vi "Main.vi"() -> ()   [LabVIEW 2019]
uses:
  Typedefs/#enum_State.ctl
  <vilib>/sound2/lvsound2.llb/Sound Data Format.ctl
  <vilib>/sound2/lvsound2.llb/Sampling Mode.ctl
  Typedefs/#cluster_ApplicationData.ctl
  <vilib>/sound2/lvsound2.llb/Sound File Refnum.ctl
  <vilib>/sound2/lvsound2.llb/Sound Input Task ID.ctl
  <vilib>/Utility/sysdir.llb/System Directory Type.ctl
  <vilib>/sound2/lvsound2.llb/Sound Input Read (DBL).vi
panel:
  out "Raw Data":waveform(dbl)[](graph)
  out "Spectrum Data":cluster{"f0":dbl, "df":dbl, "magnitude":dbl[]}[](graph)
  out "Threshold Exceeded?":bool
  in  "Threshold, dB":dbl=-100.0 format="%#_13g"
  in  "Upper Fc":dbl=3500.0 format="%#_13g"
  in  "Lower Fc":dbl=300.0 format="%#_13g"
  in  "Order":i32=6
  in  "Type":T1(ring)
  in  "Stop":bool
  # "FILTER SETTINGS"
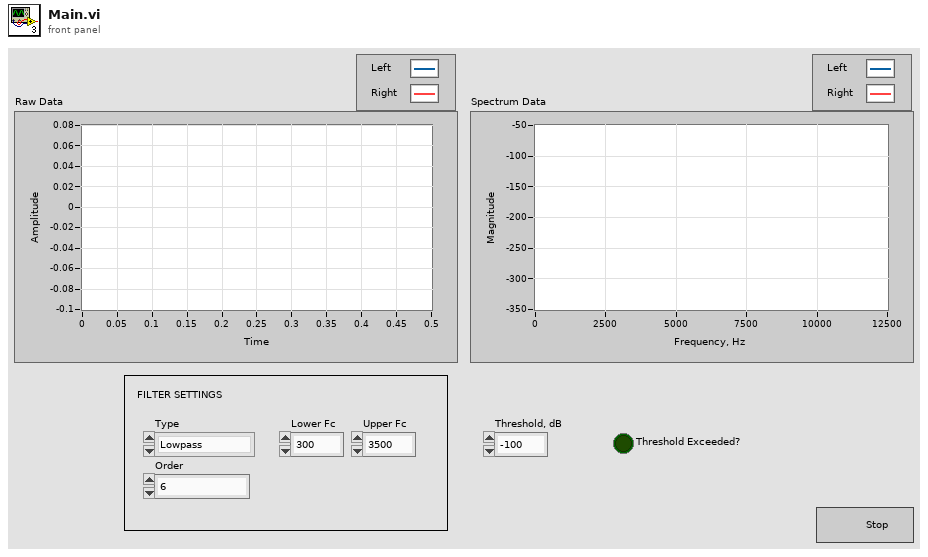
[diagram p1: front panel]
types:
  T1 = enum16{"Lowpass", "Highpass", "Bandpass", "Bandstop"}
  T2 = typedef "#enum_State.ctl" = enum16{"Init", "Acquisition", "Error Handler", "Exit"}
  T3 = enum16{"open", "replace", "create", "open or create", "replace or create", "replace or create with confirmation"}
  T4 = typedef "Sound Data Format.ctl" = cluster{"sample rate (S/s)":dbl, "number of channels":i32, "bits per sample":i32}
  T5 = typedef "#cluster_ApplicationData.ctl" = cluster{"Sound file refnum":T6, "Acquisition task ID":T7, "Sound format":T4, "Number of samples/channel":i32, "Logging file refnum":refnum<file>}
  T6 = typedef "Sound File Refnum.ctl" = refnum<file>
  T7 = typedef "Sound Input Task ID.ctl" = u32
  T8 = typedef "System Directory Type.ctl" = i32
  T9 = typedef "Sampling Mode.ctl" = i32
  T10 = cluster{"Topology":enum16{"Off", "Butterworth", "Chebyshev", "Inverse Chebyshev", "Elliptic", "Bessel"}, "Type":enum16{"Lowpass", "Highpass", "Bandpass", "Bandstop"}, "Order":i32, "Lower Fc":dbl, "Upper Fc":dbl, "PB Ripple":dbl, "SB Attenuation":dbl}
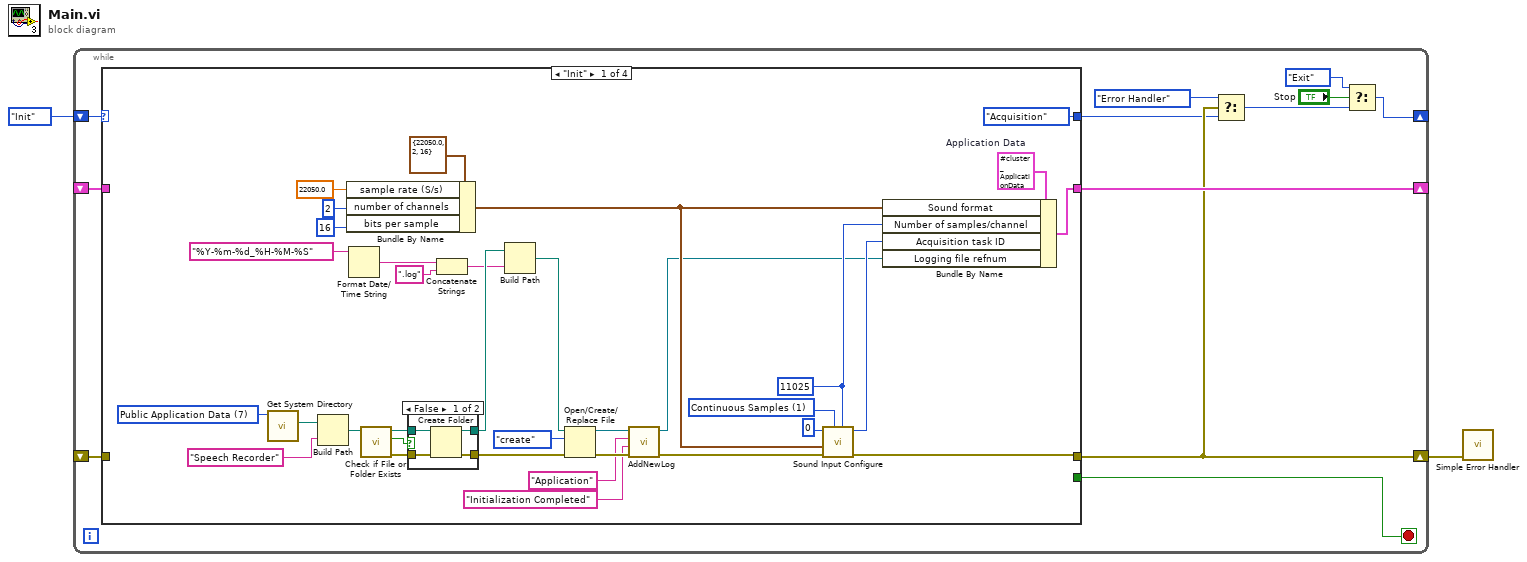
[diagram p0: block diagram]
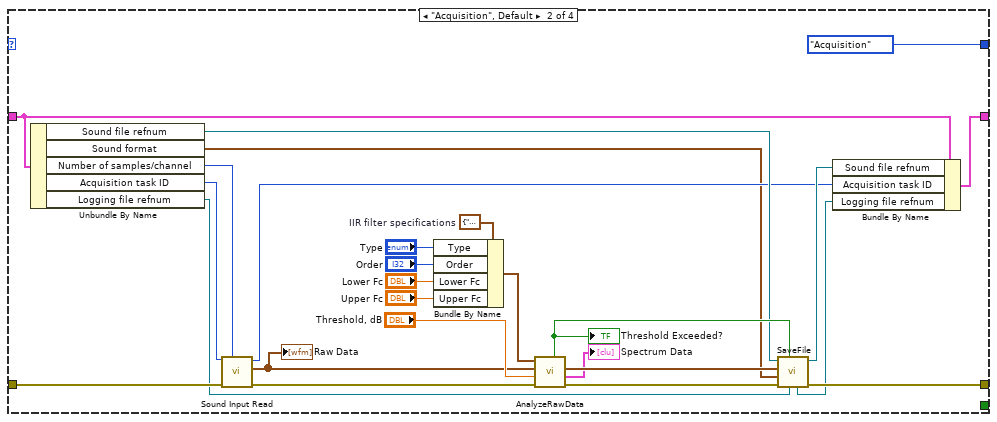
[diagram p3: hidden frame]
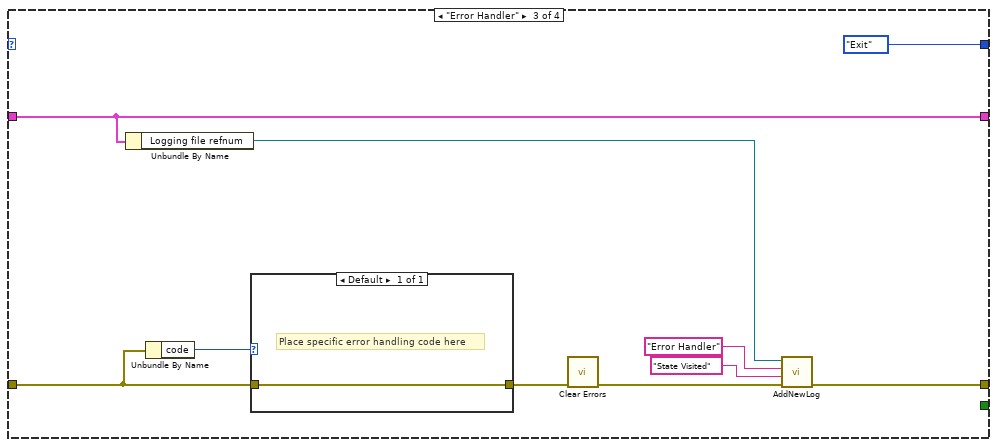
[diagram p4: hidden frame]
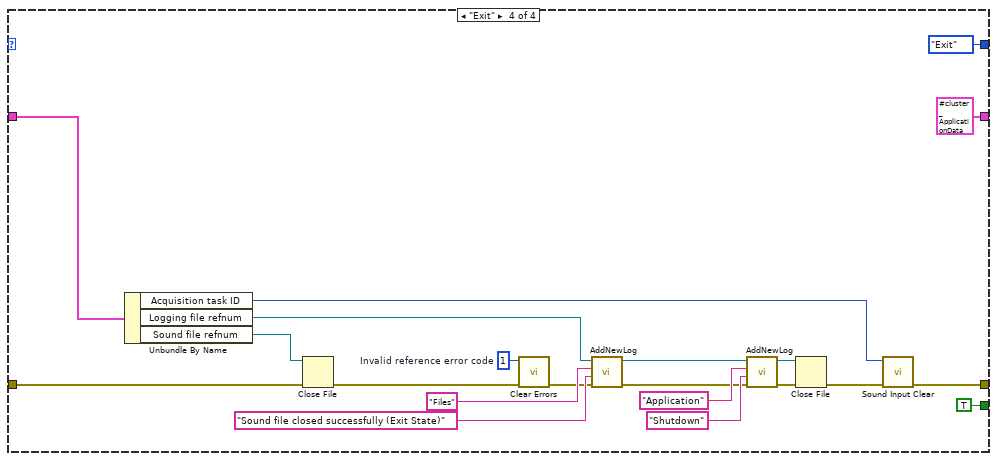
[diagram p5: hidden frame]
diagram:
  n1 = while {
    shift-right: [w5] -> _
    shift-left: #enum_State."Init" ("State") -> [w14]
    shift-right: [w12] -> _
    shift-left: _ -> [w13]
    shift-right: [w9] -> w2
    shift-left: _ -> [w11]
    stop <- w10 stop-if-true
    n2 = case shown="\"Init\"" w14 {
      tunnel: w11 -> [_ w80 w81 w112]
      tunnel: [w40 w67 w88 w95] -> w9
      tunnel: w13 -> [_ w64 w85 w109]
      tunnel: [w41 w63 w85 T5 {"Sound file refnum"=refnum, "Acquisition task ID"=0, "Sound format"={"sample rate (S/s)"=22050.0, "number of channels"=2, "bits per sample"=16}, "Number of samples/channel"=0, "Logging file refnum"=refnum} ("Application Data")] -> w12
      tunnel: [#enum_State."Acquisition" ("State") #enum_State."Acquisition" ("State") #enum_State."Exit" ("State") #enum_State."Exit" ("State")] -> w6
      tunnel: [_ _ _ TRUE] -> w10
      frame "Init" {
        w35 = T8 7 items=["User Home"=0, "User Desktop"=1, "User Documents"=2, "User Application Data"=3, "User Preferences"=4, "User Temporary"=5, "Public Documents"=6, "Public Application Data"=7, "Public Preferences"=8, "Public Cache"=13, "System Core Libraries"=9, "System Installed Libraries"=10, "Application Files"=11, "Boot Volume Root"=12] ("system directory type")
        w42 = T5 {"Sound file refnum"=refnum, "Acquisition task ID"=0, "Sound format"={"sample rate (S/s)"=22050.0, "number of channels"=2, "bits per sample"=16}, "Number of samples/channel"=0, "Logging file refnum"=refnum}  # Application Data
        w37 = 11025 ("Number of Samples/ch")
        w48 = T9 1 items=["Finite Samples", "Continuous Samples"] ("sample mode")
        n3 = call <vilib>:"Get System Directory.vi"("system directory type"=w35) -> ("system directory"=w34:path)  [unwired: 10 in]
        n4 = Build Path(base path=w34, name or relative path="Speech Recorder") -> (appended path=w32:path)
        n5 = Bundle By Name(cluster=T4 {"sample rate (S/s)"=22050.0, "number of channels"=2, "bits per sample"=16} ("sound format"), "sample rate (S/s)"=22050.0 ("Sample rate (Hz)"), "number of channels"=2 ("#Channels"), "bits per sample"=16 ("Resolution (bits)")) -> (w39:T4)
        n6 = Format Date/Time String(time format string (%c)="%Y-%m-%d_%H-%M-%S") -> (date/time string=w27:string)  [unwired: 2 in]
        n7 = call <vilib>:"Check if File or Folder Exists.vi"("path"=w32) -> ("error out"=w31:errorcluster, "file or folder exists?"=w29:bool, "dup path"=w30:path)  [unwired: 8 in]
        n8 = case shown="False" w29 {
          tunnel: w31 -> [w52 w53]
          tunnel: [w51 w53] -> w22
          tunnel: w30 -> [w50 w54]
          tunnel: [w49 w54] -> w28
          frame False {
            n9 = Create Folder(path (use dialog)=w50, error in=w52) -> (created path=w49:path, error out=w51:errorcluster)  [unwired: 1 in, 1 out]
          }
          frame True {
          }
        }
        n10 = Concatenate Strings(w27, ".log" ("string")) -> (w24:string)
        n11 = Build Path(base path=w28, name or relative path=w24) -> (appended path=w21:path)
        n12 = Open/Create/Replace File(file path (use dialog)=w21, error in=w22, operation (0:open)=T3."create") -> (refnum out=w18:refnum<file>, error out=w20:errorcluster)  [unwired: 3 in, 1 out]
        n13 = call "AddNewLog.vi"("error in"=w20, "Details"="Initialization Completed", "General Info"="Application", "Logging file refnum in"=w18) -> ("error out"=w19:errorcluster, "Logging file refnum out"=w17:refnum<file>)  [unwired: 6 in]
        n14 = call <vilib>:"Sound Input Configure.vi"("number of samples/ch"=w37, "sample mode"=w48, "error in (no error)"=w19, "sound format"=w39, "device ID"=u32 0 ("Device")) -> ("error out"=w40:errorcluster, "task ID"=w38:T7)  [unwired: 5 in]
        n15 = Bundle By Name(cluster=w42, "Sound format"=w39, "Number of samples/channel"=w37, "Acquisition task ID"=w38, "Logging file refnum"=w17) -> (w41:T5)
      }
      frame "Acquisition", Default {
        w79 = T10 {"Topology"=enum."Butterworth", "Type"=enum."Lowpass", "Order"=1, "Lower Fc"=100.0, "Upper Fc"=200.0, "PB Ripple"=1.0, "SB Attenuation"=60.0}  # IIR filter specifications
        n16 = Unbundle By Name(w64) -> ("Sound file refnum"=w65:T6, "Sound format"=w58:T4, "Number of samples/channel"=w59:i32, "Acquisition task ID"=w60:T7, "Logging file refnum"=w55:refnum<file>)
        n17 = call-poly <vilib>:"Sound Input Read.vi"("number of samples/ch"=w59, "error in (no error)"=w80, "task ID"=w60) -> ("error out"=w74:errorcluster, "data"=w72:waveform(dbl)[], "task ID out"=w61:T7)  [unwired: 6 in]
        "Raw Data" <- w72
        n18 = Bundle By Name(cluster=w79, "Type"="Type", "Order"="Order", "Lower Fc"="Lower Fc", "Upper Fc"="Upper Fc") -> (w71:T10)
        n19 = call "AnalyzeRawData.vi"("error in (no error)"=w74, "Threshold, dB"="Threshold, dB", "Raw Data"=w72, "IIR Filter Specifications"=w71) -> ("error out"=w68:errorcluster, "Power Spectrum / PSD"=→"Spectrum Data":cluster{"f0":dbl, "df":dbl, "magnitude":dbl[]}[], "Filtered Data"=w70:waveform(dbl)[], "Threshold Exceeded?"=w66:bool)  [unwired: 4 in]
        "Threshold Exceeded?" <- w66
        n20 = call "SaveFile.vi"("Logging file refnum in"=w55, "Threshold Exceeded?"=w66, "Error in"=w68, "Sound format"=w58, "Filtered Data"=w70, "Sound file refnum in"=w65) -> ("Error out"=w67:errorcluster, "Sound file refnum out"=w62:T6, "Logging file refnum out"=w56:refnum<file>)  [unwired: 3 in]
        n21 = Bundle By Name(cluster=w64, "Sound file refnum"=w62, "Acquisition task ID"=w61, "Logging file refnum"=w56) -> (w63:T5)
      }
      frame "Error Handler" {
        n22 = Unbundle By Name(w85) -> ("Logging file refnum"=w84:refnum<file>)
        n23 = Unbundle By Name(w81) -> ("code"=w83:i32)
        n24 = case shown="Default" w83 {
          tunnel: [w91] -> w82
          tunnel: w81 -> [w91]
          frame Default {
            # "Place specific error handling code here"
          }
        }
        n25 = call <vilib>:"Clear Errors.vi"("error in (no error)"=w82) -> ("error out"=w90:errorcluster)  [unwired: 5 in, 1 out]
        n26 = call "AddNewLog.vi"("error in"=w90, "Details"="State Visited" ("string"), "General Info"="Error Handler" ("string"), "Logging file refnum in"=w84) -> ("error out"=w88:errorcluster)  [unwired: 6 in, 1 out]
      }
      frame "Exit" {
        w92 = 1  # Invalid reference error code
        n27 = Unbundle By Name(w109) -> ("Acquisition task ID"=w97:T7, "Logging file refnum"=w101:refnum<file>, "Sound file refnum"=w102:T6)
        n28 = Close File(refnum=w102, error in=w112) -> (error out=w94:errorcluster)  [unwired: 1 out]
        n29 = call <vilib>:"Clear Errors.vi"("error in (no error)"=w94, "specific error code to clear (0: all)"=w92) -> ("error out"=w93:errorcluster)  [unwired: 4 in, 1 out]
        n30 = call "AddNewLog.vi"("error in"=w93, "Details"="Sound file closed successfully (Exit State)" ("string"), "General Info"="Files" ("string"), "Logging file refnum in"=w101) -> ("error out"=w103:errorcluster, "Logging file refnum out"=w100:refnum<file>)  [unwired: 6 in]
        n31 = call "AddNewLog.vi"("error in"=w103, "Details"="Shutdown" ("General Info"), "General Info"="Application", "Logging file refnum in"=w100) -> ("error out"=w107:errorcluster, "Logging file refnum out"=w106:refnum<file>)  [unwired: 6 in]
        n32 = Close File(refnum=w106, error in=w107) -> (error out=w96:errorcluster)  [unwired: 1 out]
        n33 = call <vilib>:"Sound Input Clear.vi"("error in (no error)"=w96, "task ID"=w97) -> ("error out"=w95:errorcluster)  [unwired: 9 in]
      }
    }
    n34 = Select(t=#enum_State."Error Handler" ("State"), s=w9, f=w6) -> (s? t:f=w7:T2)
    n35 = Select(t=#enum_State."Exit" ("State"), s="Stop", f=w7) -> (s? t:f=w5:T2)
  }
  n36 = call <vilib>:"Simple Error Handler.vi"("error in (no error)"=w2) -> ()  [unwired: 4 in, 5 out]
